vi "Push Waveform Batch.vi"(8 "error in (no error)":errorcluster, 10 "Waveform":waveform(dbl), 11 "Channel in":refnum<class "Channel.lvclass">) -> (0 "error out":errorcluster, 3 "Channel out":refnum<class "Channel.lvclass">)   [LabVIEW 2020, in "Nominal Streaming.lvlib" / "Channel.lvclass"]
uses:
  Channel.lvclass
  Channel.lvclass/Channel.ctl
  Stream/Stream.lvclass
  Nominal Streaming/Nominal Streaming.lvlib
  bin/lib_nominal-streaming-lv_64.dll
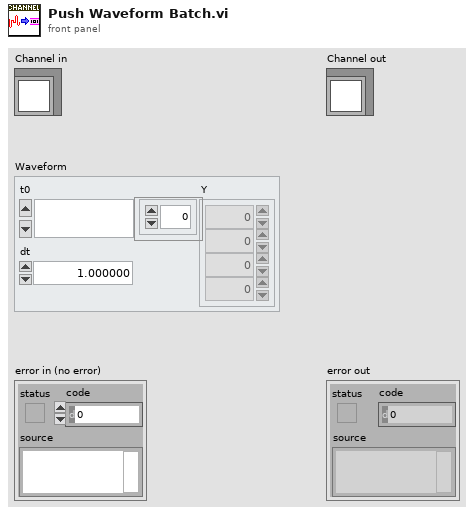
[diagram p1: front panel]
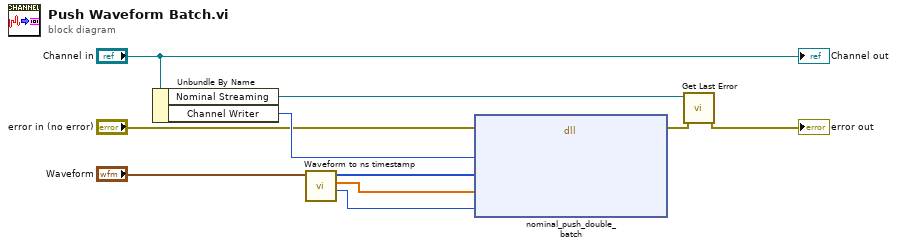
[diagram p0: block diagram]
diagram:
  n1 = Unbundle By Name("Channel in") -> ("Nominal Streaming"=w2:refnum<class "Stream.lvclass">, "Channel Writer"=w10:u64)
  n2 = call "Waveform to ns timestamp.vi"("Waveform"="Waveform") -> ("number of samples"=w3:i32, "data"=w4:dbl[], "ns timestamp"=w5:u64[])  [unwired: 8 in]
  n3 = dll-call lib="C:/code/nominal-streaming-labview-ffi/lv_src/bin/lib_nominal-streaming-lv_*.*" fn="nominal_push_double_batch"(error in="error in (no error)", "writer_handle"=w10, "timestamps_ns"=w5, "values"=w4, "count"=w3) -> (error out=w9:errorcluster)  [unwired: 7 in, 1 out]
  n4 = call "Get Last Error.vi"("error in (no error)"=w9, "Nominal Streaming in"=w2) -> ("error out"=→"error out":errorcluster)  [unwired: 8 in, 1 out]
  "Channel out" <- "Channel in"
